vi "WRITE (SubVI).vi"(10 "reference":refnum<vi>, 11 "String in":refnum<vi>) -> ()   [LabVIEW 2021]
uses:
  <vilib>/Utility/file.llb/Write Delimited Spreadsheet (string).vi
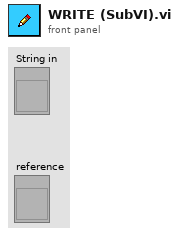
[diagram p1: front panel]
types:
  T1 = cluster{"DATE":string, "TIME":string, "NUMBER OF ROSE SOAP":dbl, "NUMBER OF LAVENDAR SOAP":dbl, "NUMBER OF STRAWBERRY SOAP":dbl, "TOTAL NUMBER OF SOAP":dbl}
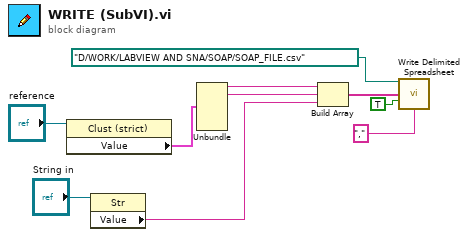
[diagram p0: block diagram]
diagram:
  n1 = property class="Clust (strict)"(reference="reference") -> ("Value"=w5:T1)  [unwired: 1 in, 2 out]
  n2 = property class="Str"(reference="String in") -> ("Value"=w8:string)  [unwired: 1 in, 2 out]
  n3 = Unbundle(w5) -> ("DATE"=w6:string, "TIME"=w7:string)  [unwired: 4 out]
  n4 = Build Array(w6, w7, w8) -> (w9:string[])
  n5 = call-poly <vilib>:"Write Delimited Spreadsheet.vi"("file path (dialog if empty)"=path "D:/WORK/LABVIEW AND SNA/SOAP/SOAP_FILE.csv", "1D data"=w9, "append to file? (new file:F)"=TRUE, "delimiter (\\t)"="," ("delimiter (\\t)")) -> ()  [unwired: 10 in, 2 out]
